vi "SetDirectTrace.vi"(8 "ErrorIn":errorcluster, 9 "TraceQueue":refnum<queue>, 11 "ObjectIn":refnum<class "TAFTraceWindow.lvclass">) -> (0 "ErrorOut":errorcluster, 3 "ObjectOut":refnum<class "TAFTraceWindow.lvclass">)   [LabVIEW 2021, in "TAFTraceWindow.lvclass"]
uses:
  TAFTraceWindow.lvclass
  TAFTraceWindow.lvclass/TAFTraceWindow.ctl
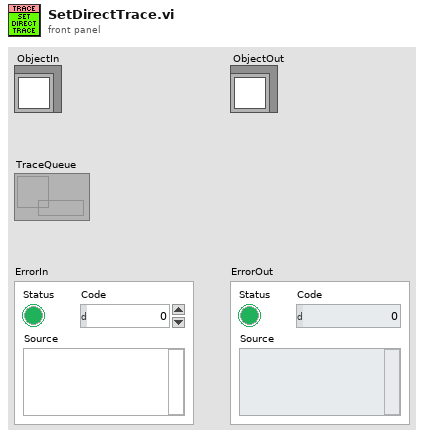
[diagram p1: front panel]
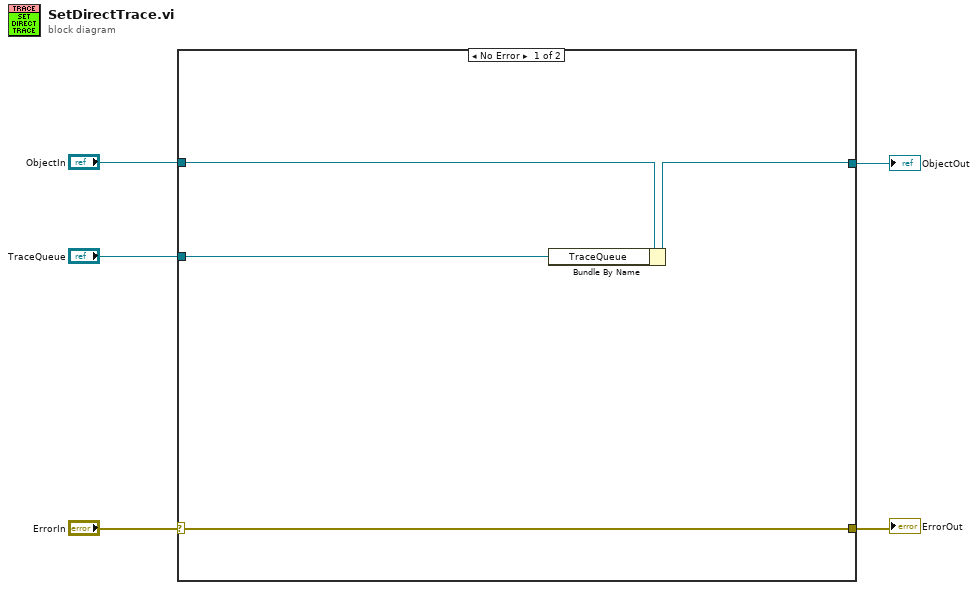
[diagram p0: block diagram]
diagram:
  n1 = case shown="No Error" "ErrorIn" {
    selector: "ErrorIn" -> [w9 w11]
    tunnel: [w9 w11] -> w4
    tunnel: [w7 w10] -> w2
    tunnel: "ObjectIn" -> [w8 w10]
    tunnel: "TraceQueue" -> [w6 _]
    frame No Error {
      n2 = Bundle By Name(cluster=w8, "TraceQueue"=w6) -> (w7:refnum<class "TAFTraceWindow.lvclass">)
    }
    frame Error {
    }
  }
  "ErrorOut" <- w4
  "ObjectOut" <- w2
